vi "Drive Controller.vi"(8 "error in":errorcluster) -> ()   [LabVIEW 2020]
doc: "This VI executes continuously carrying out the current operation and responding to updates or new operation requests. It will often contain the timing or control code that is difficult to place directly in TeleOp. This VI generally opens all sensors and motors and isolates the rest of the robot code from knowing implementation details of how the operations are carried out."
uses:
  <vilib>/Rock Robotics/WPI/Framework/Completion Status.ctl
  Drive Setpoints.ctl
  Drive Operations.ctl
  <vilib>/Rock Robotics/WPI/SafetyOutput/WPI_SafetyOutputConfigMenu.ctl
  <vilib>/Rock Robotics/WPI/ThirdParty/REV Robotics/REVLib/Typedef/Spark MAX Idle Mode.ctl
  <vilib>/Rock Robotics/WPI/RobotDrive/WPI_RobotDriveOpen2MotorWithExistingMotors.vi
  <vilib>/Rock Robotics/Network Tables/NT Write Numeric Array.vi
  <vilib>/Rock Robotics/WPI/ThirdParty/REV Robotics/REVLib/Typedef/Spark MAX Motor Type.ctl
panel:
  in  "Interactive Values":T1
  in  "Buttons":cluster{"Execute Cmd":bool, "Abort Cmd":bool}
  out "Command Timing":cluster{"Start Time (ms)":u32, "Iterations":i32}
  out "Status":T3
  out "Setpoints":T4(graph)
  out "Current\nCmd":string
  # "Tip: The graph shows the motor setpoints. It may also be helpful to observe inputs and sensor values.\nYou may also want to display tuning or debugging controls."
  # "Interactive Command: You may fill in the settings for a command\nand schedule it with the Execute button. You can observe and abort\nany command while fine tuning the code for the controller."
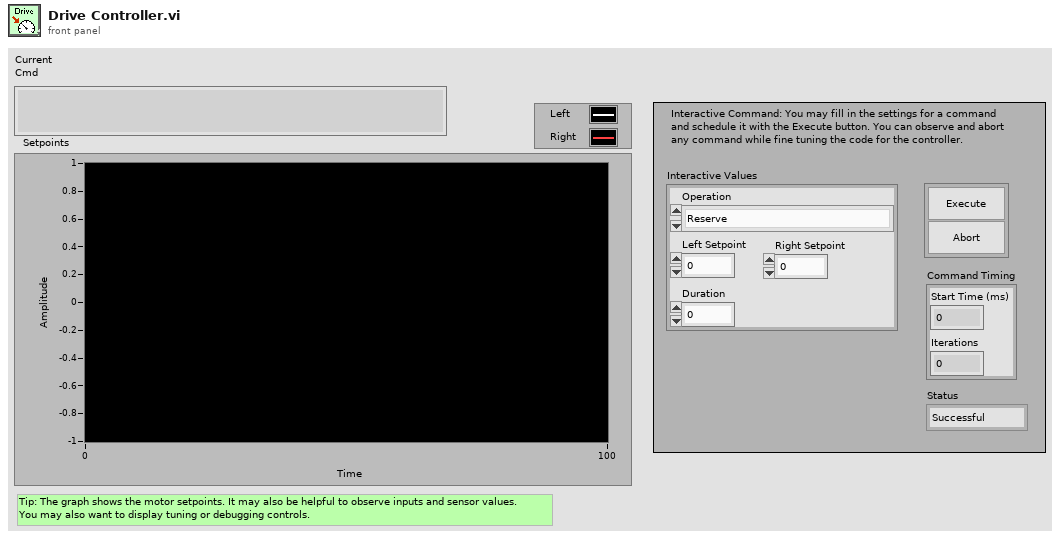
[diagram p1: front panel]
types:
  T1 = typedef "Drive Setpoints.ctl" = cluster{"Operation":T2, "Left Setpoint":dbl, "Right Setpoint":dbl, "Duration":dbl}
  T2 = typedef "Drive Operations.ctl" = enum16{"Reserve", "Read Current", "Immediate", "Drive for Time", "Drive for Distance"}
  T3 = typedef "Completion Status.ctl" = enum16{"Successful", "Aborted", "Incomplete"}
  T4 = cluster{"Left Setpoint":dbl, "Right Setpoint":dbl}
  T5 = typedef "WPI_SafetyOutputConfigMenu.ctl" = enum16{"Enable", "Disable"}
  T6 = typedef "Spark MAX Idle Mode.ctl" = enum16{"Coast", "Brake"}
  T7 = typedef "WPI_MotorControlDeviceRef.ctl" = cluster{"DeviceStatus":errorcluster, "Type":T8, "PWM":cluster{"PWM Channel":T9, "DeadBand":T10}, "CAN":cluster{"Device Number":u8, "SetOutput VI Ref":variant, "GetOutput VI Ref":variant, "Enable VI Ref":variant, "Disable VI Ref":variant, "Data":variant}, "Invert":bool, "DIO PWM":cluster{"PWM \"Enable\" Channel":T9, "DIOChannel":T11, "PWM Rate":dbl}}
  T8 = typedef "WPI_MotorControlType.ctl" = enum16{"PWM", "CAN", "DIO PWM"}
  T9 = typedef "FPGA_DIOPWMChannel.ctl" = enum8{"PWM 0", "PWM 1", "PWM 2", "PWM 3", "PWM 4", "PWM 5", "PWM 6", "PWM 7", "PWM 8", "PWM 9", "PWM MXP 0", "PWM MXP 1", "PWM MXP 2", "PWM MXP 3", "PWM MXP 4", "PWM MXP 5", "PWM MXP 6", "PWM MXP 7", "PWM MXP 8", "PWM MXP 9", "Invalid"}
  T10 = typedef "WPI_PWMDeadband.ctl" = cluster{"Name":string, "maxPositivePwm":i32, "minPositivePwm":i32, "centerPwm":i32, "maxNegativePwm":i32, "minNegativePwm":i32, "angularRange":u16}
  T11 = typedef "FPGA_DIOChannel.ctl" = enum8{"DIO 0", "DIO 1", "DIO 2", "DIO 3", "DIO 4", "DIO 5", "DIO 6", "DIO 7", "DIO 8", "DIO 9", "DIO MXP 0", "DIO MXP 1", "DIO MXP 2", "DIO MXP 3", "DIO MXP 4", "DIO MXP 5", "DIO MXP 6", "DIO MXP 7", "DIO MXP 8", "DIO MXP 9", "DIO MXP 10", "DIO MXP 11", "DIO MXP 12", "DIO MXP 13", "DIO MXP 14", "DIO MXP 15", "SPI Port CS1", "SPI Port CS2", "SPI Port CS3", "SPI Port MISO", "SPI Port MOSI", "Invalid"}
  T12 = typedef "Spark MAX Motor Type.ctl" = enum16{"Brushed", "Brushless"}
  T13 = typedef "WPI_RobotDriveDevRef.ctl" = cluster{"DevStatus":errorcluster, "Motors[]":T7[], "Square Inputs":bool, "Max Output":dbl}
  T14 = typedef "Command Status Info.ctl" = cluster{"Name":string, "Status":T3, "notifier out":T15}
  T15 = typedef "Completion Notifier.ctl" = refnum<notifier>
  T16 = cluster{"SubSystem Data":T1, cluster{"Start Time (ms)":u32, "Iterations":i32}, cluster{"Command Info":T14, "Description":string, "Default Command":T1, "queue out":refnum<queue>, "Subsystem Name":string}}
  T17 = cluster{"SubSystem Data":T1, cluster{"Start Time (ms)":u32, "Iterations":i32}, "Default Command Arguments":cluster{"Command Info":T14, "Description":string, "Default Command":T1, "queue out":refnum<queue>, "Subsystem Name":string}}
  T18 = cluster{"Don't move motors while reserved":dbl, "Don't move motors while reserved":dbl}
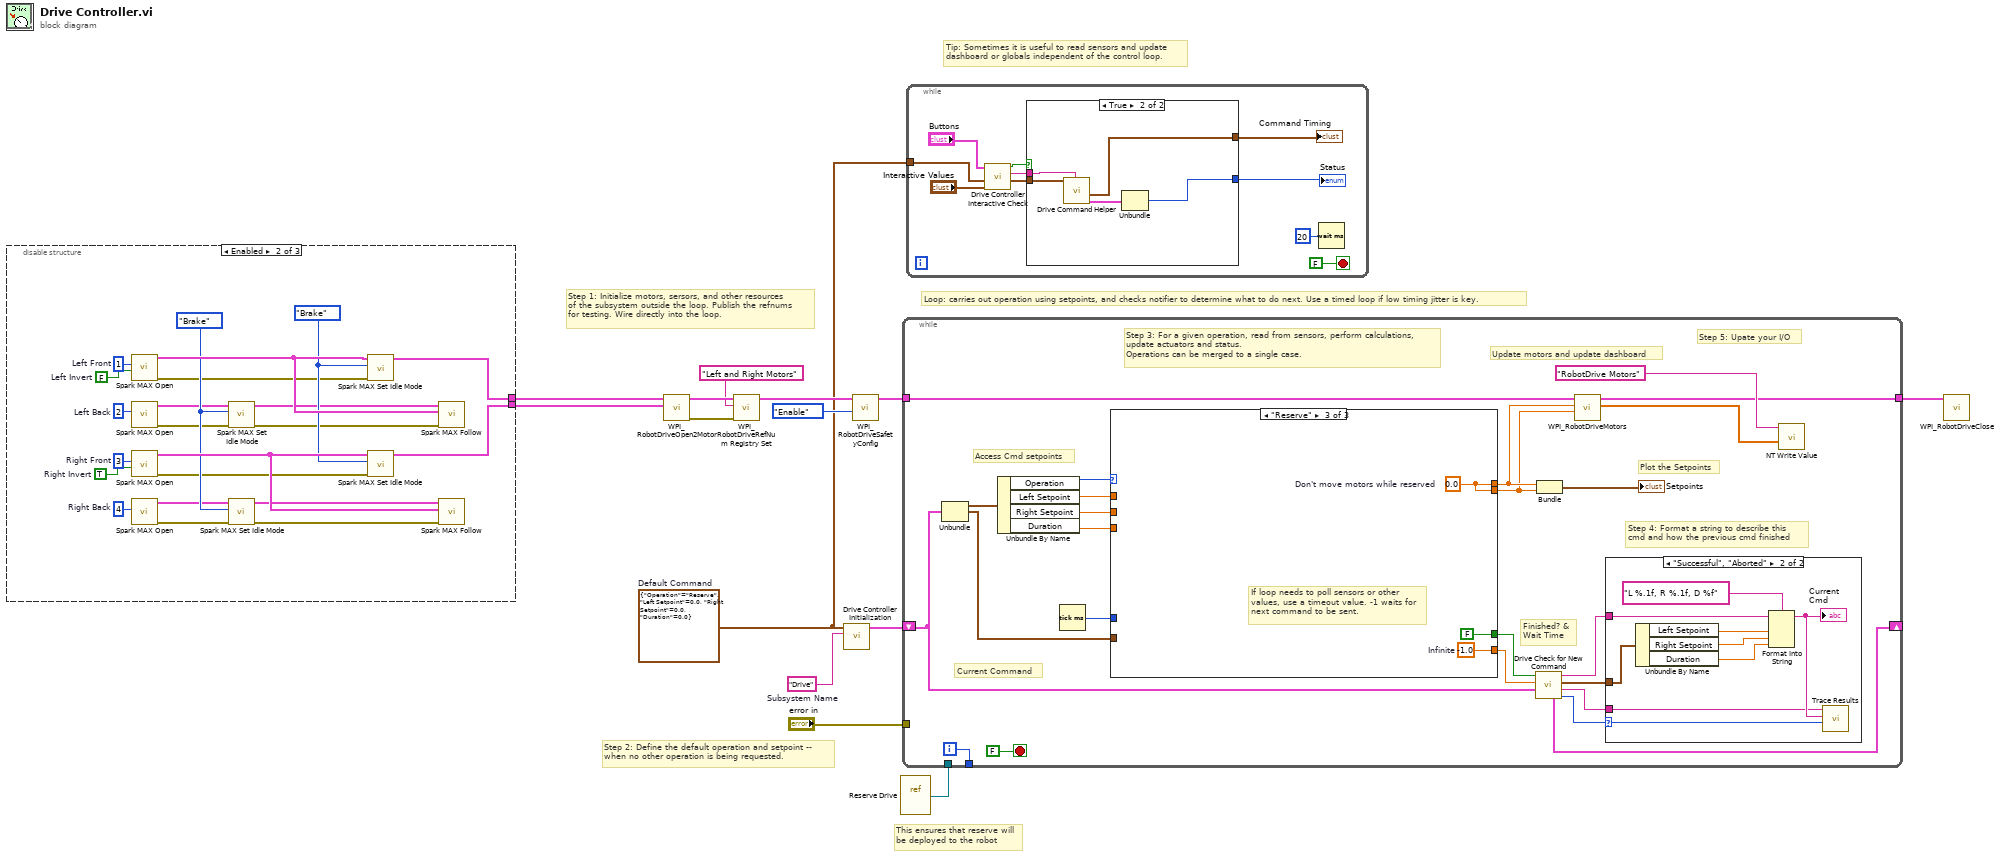
[diagram p0: block diagram]
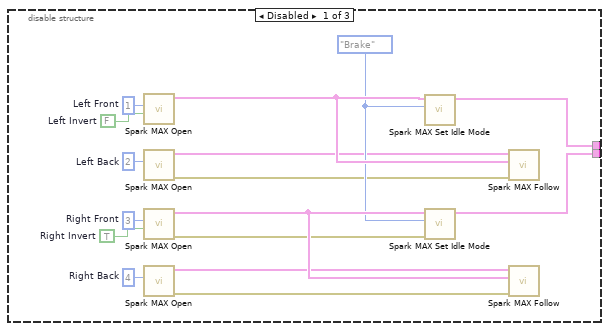
[diagram p2: hidden frame]
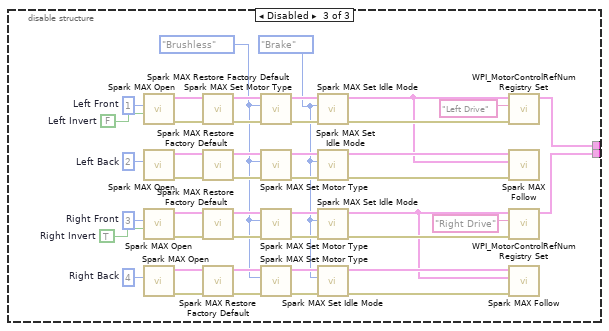
[diagram p3: hidden frame]
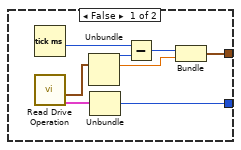
[diagram p4: hidden frame]
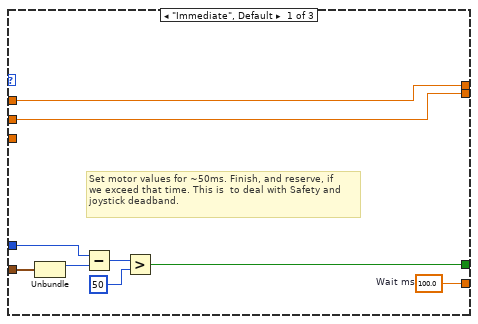
[diagram p6: hidden frame]
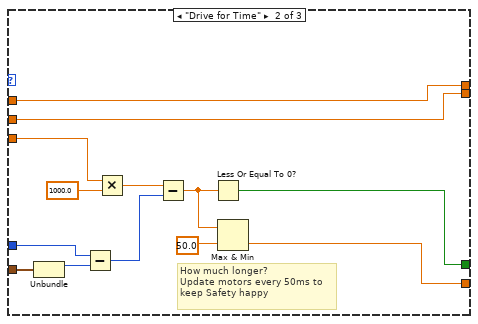
[diagram p7: hidden frame]
diagram:
  w4 = T1 {"Operation"=enum."Reserve", "Left Setpoint"=0.0, "Right Setpoint"=0.0, "Duration"=0.0}  # Default Command
  w14 = "Drive"  # Subsystem Name
  # "This ensures that reserve will\nbe deployed to the robot"
  # "Tip: Sometimes it is useful to read sensors and update\ndashboard or globals independent of the control loop."
  # "Step 2: Define the default operation and setpoint --\nwhen no other operation is being requested."
  # "Step 1: Initialize motors, sersors, and other resources\nof the subsystem outside the loop. Publish the refnums\nfor testing. Wire directly into the loop."
  # "Loop: carries out operation using setpoints, and checks notifier to determine what to do next. Use a timed loop if low timing jitter is key."
  n1 = disable-structure shown="Enabled" {
    disable-tunnel: [w23 w45 w56] -> w3
    disable-tunnel: [w21 w43 w55] -> w2
    frame Disabled {
      w20 = Spark_MAX_Idle_Mode."Brake" ("Idle Mode")
      w25 = u8 4  # Right Back
      w26 = u8 3  # Right Front
      w27 = u8 2  # Left Back
      w28 = u8 1  # Left Front
      w29 = TRUE  # Right Invert
      w30 = FALSE  # Left Invert
      n2 = call <vilib>:"Spark MAX Open.vi"("Invert"=w30, "Device Number"=w28) -> ("MotorControlDeviceRef"=w24:T7)  [unwired: 8 in, 1 out]
      n3 = call <vilib>:"Spark MAX Open.vi"("Device Number"=w27) -> ("error out"=w18:errorcluster, "MotorControlDeviceRef"=w19:T7)  [unwired: 9 in]
      n4 = call <vilib>:"Spark MAX Open.vi"("Invert"=w29, "Device Number"=w26) -> ("error out"=w17:errorcluster, "MotorControlDeviceRef"=w22:T7)  [unwired: 8 in]
      n5 = call <vilib>:"Spark MAX Open.vi"("Device Number"=w25) -> ("error out"=w15:errorcluster, "MotorControlDeviceRef"=w16:T7)  [unwired: 9 in]
      n6 = call <vilib>:"Spark MAX Set Idle Mode.vi"("Idle Mode"=w20, "MotorControlDeviceRef in"=w24) -> ("MotorControlDeviceRef out"=w23:T7)  [unwired: 8 in, 1 out]
      n7 = call <vilib>:"Spark MAX Set Idle Mode.vi"("error in (no error)"=w17, "Idle Mode"=w20, "MotorControlDeviceRef in"=w22) -> ("MotorControlDeviceRef out"=w21:T7)  [unwired: 7 in, 1 out]
      n8 = call <vilib>:"Spark MAX Follow.vi"("error in (no error)"=w18, "Master Controller"=w24, "MotorControlDeviceRef"=w19) -> ()  [unwired: 7 in, 2 out]
      n9 = call <vilib>:"Spark MAX Follow.vi"("error in (no error)"=w15, "Master Controller"=w22, "MotorControlDeviceRef"=w16) -> ()  [unwired: 7 in, 2 out]
    }
    frame Enabled {
      w41 = Spark_MAX_Idle_Mode."Brake" ("Idle Mode")
      w42 = Spark_MAX_Idle_Mode."Brake" ("Idle Mode")
      w47 = u8 4  # Right Back
      w48 = u8 3  # Right Front
      w49 = u8 2  # Left Back
      w50 = u8 1  # Left Front
      w51 = TRUE  # Right Invert
      w52 = FALSE  # Left Invert
      n10 = call <vilib>:"Spark MAX Open.vi"("Invert"=w52, "Device Number"=w50) -> ("error out"=w31:errorcluster, "MotorControlDeviceRef"=w46:T7)  [unwired: 8 in]
      n11 = call <vilib>:"Spark MAX Open.vi"("Device Number"=w49) -> ("error out"=w38:errorcluster, "MotorControlDeviceRef"=w40:T7)  [unwired: 9 in]
      n12 = call <vilib>:"Spark MAX Open.vi"("Invert"=w51, "Device Number"=w48) -> ("error out"=w36:errorcluster, "MotorControlDeviceRef"=w44:T7)  [unwired: 8 in]
      n13 = call <vilib>:"Spark MAX Open.vi"("Device Number"=w47) -> ("error out"=w33:errorcluster, "MotorControlDeviceRef"=w35:T7)  [unwired: 9 in]
      n14 = call <vilib>:"Spark MAX Set Idle Mode.vi"("error in (no error)"=w38, "Idle Mode"=w41, "MotorControlDeviceRef in"=w40) -> ("error out"=w37:errorcluster, "MotorControlDeviceRef out"=w39:T7)  [unwired: 7 in]
      n15 = call <vilib>:"Spark MAX Set Idle Mode.vi"("error in (no error)"=w33, "Idle Mode"=w41, "MotorControlDeviceRef in"=w35) -> ("error out"=w32:errorcluster, "MotorControlDeviceRef out"=w34:T7)  [unwired: 7 in]
      n16 = call <vilib>:"Spark MAX Set Idle Mode.vi"("error in (no error)"=w31, "Idle Mode"=w42, "MotorControlDeviceRef in"=w46) -> ("MotorControlDeviceRef out"=w45:T7)  [unwired: 7 in, 1 out]
      n17 = call <vilib>:"Spark MAX Set Idle Mode.vi"("error in (no error)"=w36, "Idle Mode"=w42, "MotorControlDeviceRef in"=w44) -> ("MotorControlDeviceRef out"=w43:T7)  [unwired: 7 in, 1 out]
      n18 = call <vilib>:"Spark MAX Follow.vi"("error in (no error)"=w37, "Master Controller"=w46, "MotorControlDeviceRef"=w39) -> ()  [unwired: 7 in, 2 out]
      n19 = call <vilib>:"Spark MAX Follow.vi"("error in (no error)"=w32, "Master Controller"=w44, "MotorControlDeviceRef"=w34) -> ()  [unwired: 7 in, 2 out]
    }
    frame Disabled {
      w53 = Spark_MAX_Idle_Mode."Brake" ("Idle Mode")
      w54 = Spark_MAX_Motor_Type."Brushless" ("Motor Type")
      w63 = u8 4  # Right Back
      w64 = u8 3  # Right Front
      w65 = u8 2  # Left Back
      w66 = u8 1  # Left Front
      w67 = TRUE  # Right Invert
      w68 = FALSE  # Left Invert
      n20 = call <vilib>:"Spark MAX Open.vi"("Invert"=w68, "Device Number"=w66) -> ("error out"=w96:errorcluster, "MotorControlDeviceRef"=w95:T7)  [unwired: 8 in]
      n21 = call <vilib>:"Spark MAX Open.vi"("Device Number"=w65) -> ("error out"=w85:errorcluster, "MotorControlDeviceRef"=w86:T7)  [unwired: 9 in]
      n22 = call <vilib>:"Spark MAX Open.vi"("Invert"=w67, "Device Number"=w64) -> ("error out"=w79:errorcluster, "MotorControlDeviceRef"=w80:T7)  [unwired: 8 in]
      n23 = call <vilib>:"Spark MAX Open.vi"("Device Number"=w63) -> ("error out"=w74:errorcluster, "MotorControlDeviceRef"=w73:T7)  [unwired: 9 in]
      n24 = call <vilib>:"Spark MAX Restore Factory Default.vi"("error in"=w96, "MotorControlDeviceRef"=w95) -> ("error out"=w94:errorcluster, "MotorControlDeviceRef"=w93:T7)  [unwired: 8 in]
      n25 = call <vilib>:"Spark MAX Restore Factory Default.vi"("error in"=w85, "MotorControlDeviceRef"=w86) -> ("error out"=w87:errorcluster, "MotorControlDeviceRef"=w88:T7)  [unwired: 8 in]
      n26 = call <vilib>:"Spark MAX Restore Factory Default.vi"("error in"=w79, "MotorControlDeviceRef"=w80) -> ("error out"=w81:errorcluster, "MotorControlDeviceRef"=w82:T7)  [unwired: 8 in]
      n27 = call <vilib>:"Spark MAX Restore Factory Default.vi"("error in"=w74, "MotorControlDeviceRef"=w73) -> ("error out"=w72:errorcluster, "MotorControlDeviceRef"=w71:T7)  [unwired: 8 in]
      n28 = call <vilib>:"Spark MAX Set Motor Type.vi"("error in (no error)"=w94, "Motor Type"=w54, "MotorControlDevRef"=w93) -> ("error out"=w92:errorcluster, "MotorControlDeviceRef"=w91:T7)  [unwired: 7 in]
      n29 = call <vilib>:"Spark MAX Set Motor Type.vi"("error in (no error)"=w87, "Motor Type"=w54, "MotorControlDevRef"=w88) -> ("error out"=w89:errorcluster, "MotorControlDeviceRef"=w90:T7)  [unwired: 7 in]
      n30 = call <vilib>:"Spark MAX Set Motor Type.vi"("error in (no error)"=w81, "Motor Type"=w54, "MotorControlDevRef"=w82) -> ("error out"=w83:errorcluster, "MotorControlDeviceRef"=w84:T7)  [unwired: 7 in]
      n31 = call <vilib>:"Spark MAX Set Motor Type.vi"("error in (no error)"=w72, "Motor Type"=w54, "MotorControlDevRef"=w71) -> ("error out"=w70:errorcluster, "MotorControlDeviceRef"=w69:T7)  [unwired: 7 in]
      n32 = call <vilib>:"Spark MAX Set Idle Mode.vi"("error in (no error)"=w92, "Idle Mode"=w53, "MotorControlDeviceRef in"=w91) -> ("error out"=w62:errorcluster, "MotorControlDeviceRef out"=w60:T7)  [unwired: 7 in]
      n33 = call <vilib>:"Spark MAX Set Idle Mode.vi"("error in (no error)"=w89, "Idle Mode"=w53, "MotorControlDeviceRef in"=w90) -> ("error out"=w78:errorcluster, "MotorControlDeviceRef out"=w77:T7)  [unwired: 7 in]
      n34 = call <vilib>:"Spark MAX Set Idle Mode.vi"("error in (no error)"=w83, "Idle Mode"=w53, "MotorControlDeviceRef in"=w84) -> ("error out"=w61:errorcluster, "MotorControlDeviceRef out"=w59:T7)  [unwired: 7 in]
      n35 = call <vilib>:"Spark MAX Set Idle Mode.vi"("error in (no error)"=w70, "Idle Mode"=w53, "MotorControlDeviceRef in"=w69) -> ("error out"=w75:errorcluster, "MotorControlDeviceRef out"=w76:T7)  [unwired: 7 in]
      n36 = call <vilib>:"WPI_MotorControlRefNum Registry Set.vi"("error in (no error)"=w62, "refnum name"="Left Drive", "MotorControlDevRef"=w60) -> ("MotorControlDevRef"=w56:T7)  [unwired: 7 in, 1 out]
      n37 = call <vilib>:"Spark MAX Follow.vi"("error in (no error)"=w78, "Master Controller"=w60, "MotorControlDeviceRef"=w77) -> ()  [unwired: 7 in, 2 out]
      n38 = call <vilib>:"WPI_MotorControlRefNum Registry Set.vi"("error in (no error)"=w61, "refnum name"="Right Drive", "MotorControlDevRef"=w59) -> ("MotorControlDevRef"=w55:T7)  [unwired: 7 in, 1 out]
      n39 = call <vilib>:"Spark MAX Follow.vi"("error in (no error)"=w75, "Master Controller"=w59, "MotorControlDeviceRef"=w76) -> ()  [unwired: 7 in, 2 out]
    }
  }
  n40 = call-poly <vilib>:"WPI_RobotDriveOpen2Motor.vi"("Right Motor Dev Ref"=w2, "Left Motor Dev Ref"=w3) -> ("error out"=w11:errorcluster, "RobotDriveDevRef"=w13:T13)  [unwired: 3 in, 5 out]
  n41 = call <vilib>:"WPI_RobotDriveRefNum Registry Set.vi"("error in (no error)"=w11, "refnum name"="Left and Right Motors", "RobotDriveDevRef"=w13) -> ("RobotDriveDevRef"=w10:T13)  [unwired: 1 in, 7 out]
  n42 = call "Drive Controller Initialization.vi"("Subsystem Name"=w14, "Default Command"=w4) -> ("Current Command"=w6:T16)  [unwired: 9 in]
  n43 = call <vilib>:"WPI_RobotDriveSafetyConfig.vi"("mode"=WPI_SafetyOutputConfigMenu."Enable", "RobotDriveDevRef"=w10) -> ("RobotDriveDevRef"=w8:T13)  [unwired: 8 in, 1 out]
  n44 = vi-ref "Reserve Drive.vi"() -> (w5:refnum<vi>)
  n45 = while {
    shift-right: [w107] -> _
    shift-left: w6 -> [w100]
    tunnel: [w119] -> _
    tunnel: w8 -> [w115]
    tunnel: "error in" -> [_]
    tunnel: w5 -> [_]
    tunnel: [w97] -> w1
    i -> [w119]
    stop <- FALSE stop-if-true
    # "Step 5: Upate your I/O"
    # "Step 4: Format a string to describe this\ncmd and how the previous cmd finished"
    # "Current Command"
    # "Update motors and update dashboard"
    # "Plot the Setpoints"
    # "Access Cmd setpoints"
    # "Finished? &\nWait Time"
    # "Step 3: For a given operation, read from sensors, perform calculations,\nupdate actuators and status.\nOperations can be merged to a single case."
    n46 = Unbundle(w100) -> ("SubSystem Data"=w114:T1, w101:cluster{"Start Time (ms)":u32, "Iterations":i32})  [unwired: 1 out]
    n47 = Unbundle By Name(w114) -> ("Operation"=w113:T2, "Left Setpoint"=w112:dbl, "Right Setpoint"=w111:dbl, "Duration"=w110:dbl)
    n48 = Tick Count (ms)() -> (millisecond timer value=w109:u32)
    n49 = case shown="\"Reserve\"" w113 {
      tunnel: [w138 w139 w154] -> w106
      tunnel: [w131 w146 FALSE ("ignore previous (F)")] -> w105
      tunnel: w101 -> [w130 w148 _]
      tunnel: [w137 w145 w152] -> w117
      tunnel: [w136 w144 w152] -> w116
      tunnel: w112 -> [w137 w145 _]
      tunnel: w111 -> [w136 w144 _]
      tunnel: w110 -> [_ w143 _]
      tunnel: w109 -> [w132 w142 _]
      frame "Immediate", Default {
        w138 = 100.0  # Wait ms
        # "Set motor values for ~50ms. Finish, and reserve, if\nwe exceed that time. This is  to deal with Safety and\njoystick deadband."
        n50 = Unbundle(w130) -> ("Start Time (ms)"=w133:u32)  [unwired: 1 out]
        n51 = Subtract(x=w132, y=w133) -> (x-y=w134:u32)
        n52 = Greater?(x=w134, y=u8 50 ("Left Motor")) -> (0:w131:bool)
      }
      frame "Drive for Time" {
        # "How much longer?\nUpdate motors every 50ms to\nkeep Safety happy"
        n53 = Unbundle(w148) -> ("Start Time (ms)"=w147:u32)  [unwired: 1 out]
        n54 = Subtract(x=w142, y=w147) -> (x-y=w151:u32)
        n55 = Multiply(x=w143, y=1000.0) -> (x*y=w150:dbl)
        n56 = Subtract(x=w150, y=w151) -> (x-y=w141:dbl)
        n57 = Less Or Equal To 0?(x=w141) -> (x <= 0?=w146:bool)
        n58 = Max & Min(x=w141, y=50.0) -> (min(x,y)=w139:dbl)  [unwired: 1 out]
      }
      frame "Reserve" {
        w152 = 0.0  # Don't move motors while reserved
        w154 = -1.0  # Infinite
        # "If loop needs to poll sensors or other\nvalues, use a timeout value. -1 waits for\nnext command to be sent."
      }
    }
    n59 = call "Drive Check for New Command.vi"("input cluster"=w100, "Wait time (ms)"=w106, "Finished?"=w105) -> ("Completion"=w108:T3, "Subsystem Name"=w102:string, "Current Command"=w103:T1, "Initial Trace String"=w104:string, "Next Command"=w107:T17)  [unwired: 4 in]
    n60 = Bundle("Don't move motors while reserved"=w117, "Don't move motors while reserved"=w116) -> (→"Setpoints":T18)  [unwired: 1 in]
    n61 = call <vilib>:"WPI_RobotDriveMotors.vi"("RightSpeed"=w116, "LeftSpeed"=w117, "RobotDriveDevRef"=w115) -> ("Motor Values"=w98:dbl[], "RobotDriveDevRef"=w97:T13)  [unwired: 1 in, 6 out]
    n62 = case shown="\"Successful\", \"Aborted\"" w108 {
      selector: w108 -> [_ w129]
      tunnel: w104 -> [_ w124]
      tunnel: w103 -> [_ w125]
      tunnel: w102 -> [_ w121]
      frame "Incomplete", Default {
        # "Continuing current command"
      }
      frame "Successful", "Aborted" {
        # "Report and setup for next command"
        n63 = Unbundle By Name(w125) -> ("Left Setpoint"=w127:dbl, "Right Setpoint"=w128:dbl, "Duration"=w122:dbl)
        n64 = Format Into String(format string="L %.1f, R %.1f, D %f", initial string=w124, w127, w128, w122) -> (resulting string=w123:string)  [unwired: 1 in, 1 out]
        "Current\nCmd" <- w123
        n65 = call <vilib>:"Trace Results.vi"("Status of previous command"=w129, "Description"=w123, "Subsystem"=w121) -> ()  [unwired: 9 in]
      }
    }
    n66 = call-poly <vilib>:"NT Write Value.vi"("Numeric Array"=w98, "Name"="RobotDrive Motors") -> ()  [unwired: 9 in, 1 out]
  }
  n67 = while {
    tunnel: w4 -> [w156]
    stop <- FALSE stop-if-true
    n68 = call "Drive Controller Interactive Check.vi"("Interactive Command In"="Interactive Values", "Default Command"=w156, "Buttons"="Buttons") -> ("Interactive Command Out"=w158:T1, "Trace String"=w159:string, "Schedule"=w160:bool)  [unwired: 6 in]
    n69 = case shown="True" w160 {
      tunnel: [w169 w177] -> w161
      tunnel: [w168 w173] -> w162
      tunnel: w159 -> [_ w175]
      tunnel: w158 -> [_ w174]
      frame False {
        n70 = Tick Count (ms)() -> (millisecond timer value=w172:u32)
        n71 = call "Read Drive Operation.vi"() -> ("Command Info"=w166:T14, "SubSystem Data"=w165:T1)  [unwired: 9 in, 1 out]
        n72 = Unbundle(w165) -> ("Operation"=w170:T2, "Left Setpoint"=w167:dbl)  [unwired: 2 out]
        n73 = Unbundle(w166) -> ("Status"=w169:T3)  [unwired: 2 out]
        n74 = Subtract(x=w172, y=w170) -> (x-y=w171:u32)
        n75 = Bundle(w171, "Left Setpoint"=w167) -> (w168:cluster{u32, "Left Setpoint":dbl})  [unwired: 1 in]
      }
      frame True {
        n76 = call "Drive Command Helper.vi"("Description"=w175, "SubSystem Data"=w174) -> ("Command Info Out"=w176:T14, "Command Timing"=w173:cluster{"Start Time (ms)":u32, "Iterations":i32})  [unwired: 7 in, 1 out]
        n77 = Unbundle(w176) -> ("Status"=w177:T3)  [unwired: 2 out]
      }
    }
    "Status" <- w161
    "Command Timing" <- w162
    n78 = Wait (ms)(milliseconds to wait=u32 20) -> ()  [unwired: 1 out]
  }
  n79 = call <vilib>:"WPI_RobotDriveClose.vi"("RobotDriveDevRef"=w1) -> ()  [unwired: 10 in, 1 out]
